vi "Servo MSMT NR Set DC Params.vi"(8 "error in (no error)":errorcluster, 10 "Step In":refnum<k7>, 11 "Servo MSMT in":refnum<class "Servo MSMT.lvclass">) -> (0 "error out":errorcluster, 2 "Step Out":refnum<k7>, 3 "Servo MSMT out":refnum<class "Servo MSMT.lvclass">)   [LabVIEW 2018, in "Servo MSMT.lvlib" / "Servo MSMT.lvclass"]
uses:
  Servo MSMT.lvclass
  Servo MSMT.lvclass/Servo MSMT.ctl
  Protected Methods/Read DC Pins.vi
  Protected Methods/Read PAE Pins.vi
  Protected Methods/Read PAE Enable Override_.vi
  Plugins/TestStand API Tools (TSAT).lvlibp/Step Actions/TSAT Step Actions.lvlib
  Plugins/Measurement Interface.lvlibp/Measurement Interface.lvclass
  C:/Sequence Automation/Plugins/Measurement Interface.lvlibp/Measurement Interface.lvclass
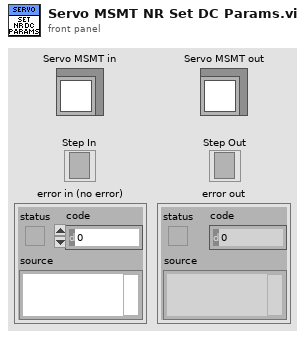
[diagram p1: front panel]
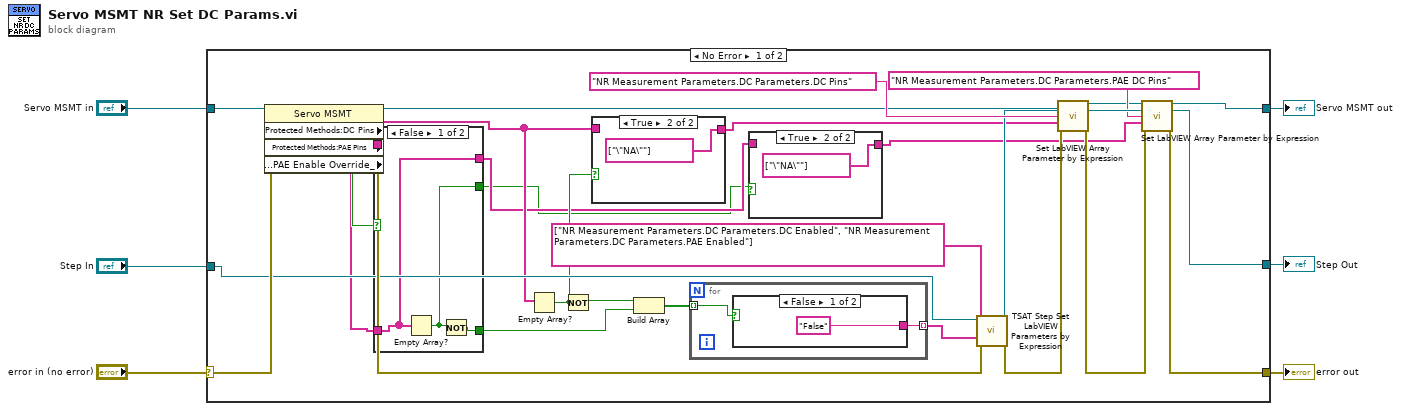
[diagram p0: block diagram]
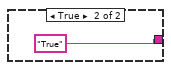
[diagram p2: hidden frame]
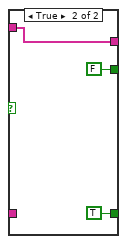
[diagram p3: hidden frame]
diagram:
  n1 = case shown="No Error" "error in (no error)" {
    selector: "error in (no error)" -> [w34 w51]
    tunnel: [w30 w51] -> w5
    tunnel: [w24 w50] -> w3
    tunnel: "Servo MSMT in" -> [w33 w50]
    tunnel: "Step In" -> [w21 w49]
    tunnel: [w28 w49] -> w1
    frame No Error {
      n2 = property class="Servo MSMT"(reference=w33, error in=w34) -> (reference out=w26:refnum<class "Servo MSMT.lvclass">, error out=w23:errorcluster, "Protected Methods:DC Pins"=w15:string[], "Protected Methods:PAE Pins"=w14:string[], "Protected Methods:PAE Enable Override_"=w16:bool)
      n3 = case shown="False" w16 {
        tunnel: w15 -> [_ w44]
        tunnel: w14 -> [w40 _]
        tunnel: [w41 TRUE] -> w13
        tunnel: [w40 w44] -> w8
        tunnel: [w39 FALSE ("empty?")] -> w7
        frame False {
          n4 = Empty Array?(array=w40) -> (empty?=w39:bool)
          n5 = Not(x=w39) -> (.not. x?=w41:bool)
        }
        frame True {
        }
      }
      n6 = Empty Array?(array=w15) -> (empty?=w19:bool)
      n7 = Not(x=w19) -> (.not. x?=w9:bool)
      n8 = case shown="True" w19 {
        tunnel: w15 -> [w47 _]
        tunnel: [w47 string[] ["\"NA\""] ("Protected Methods:DC Pins")] -> w18
        frame False {
        }
        frame True {
        }
      }
      n9 = Build Array(w9, w13) -> (w12:bool[])
      n10 = for {
        tunnel: w12 -> [w36] mode=indexing
        tunnel: [w35] -> w11 mode=indexing
        n11 = case shown="False" w36 {
          tunnel: ["False" "True"] -> w35
          frame False {
          }
          frame True {
          }
        }
      }
      n12 = case shown="True" w7 {
        tunnel: w8 -> [w45 _]
        tunnel: [w45 string[] ["\"NA\""] ("Protected Methods:DC Pins")] -> w17
        frame False {
        }
        frame True {
        }
      }
      n13 = call "TSAT Step Set LabVIEW Parameters by Expression.vi"("Error In"=w23, "Value Expressions"=w11, "Parameters to Set"=string[] ["NR Measurement Parameters.DC Parameters.DC Enabled", "NR Measurement Parameters.DC Parameters.PAE Enabled"], "Step In"=w21) -> ("Error Out"=w22:errorcluster, "Step Out"=w20:refnum<k7>)  [unwired: 6 in]
      n14 = call "Set LabVIEW Array Parameter by Expression.vi"("Measurement Interface in"=w26, "Step In"=w20, "LabVIEW Parameter to Set"="NR Measurement Parameters.DC Parameters.DC Pins", "Array of Expresssions"=w18, "error in (no error)"=w22) -> ("Measurement Interface out"=w25:refnum<class "Servo MSMT.lvclass">, "Step Out"=w29:refnum<k7>, "error out"=w31:errorcluster)  [unwired: 8 in]
      n15 = call "Set LabVIEW Array Parameter by Expression.vi"("Measurement Interface in"=w25, "Step In"=w29, "LabVIEW Parameter to Set"="NR Measurement Parameters.DC Parameters.PAE DC Pins", "Array of Expresssions"=w17, "error in (no error)"=w31) -> ("Measurement Interface out"=w24:refnum<class "Servo MSMT.lvclass">, "Step Out"=w28:refnum<k7>, "error out"=w30:errorcluster)  [unwired: 8 in]
    }
    frame Error {
    }
  }
  "error out" <- w5
  "Servo MSMT out" <- w3
  "Step Out" <- w1
